vi "ImageFileOpenwithIMAQ-U16.vi"(1 "type":u32, 2 "image filepath":path=path "I:/160830- miura/20 um beads/nonsheet/160903/test2_00004.png") -> (0 "output array":u16[][](array[numeric]))   [LabVIEW 2018]
uses:
  <vilib>/Utility/file.llb/Read Delimited Spreadsheet (DBL).vi
panel:
  out "file path for TPEF 2":path=path "C:/Users/Mikami/Desktop/test.bmp"
  out "result string":string="png"
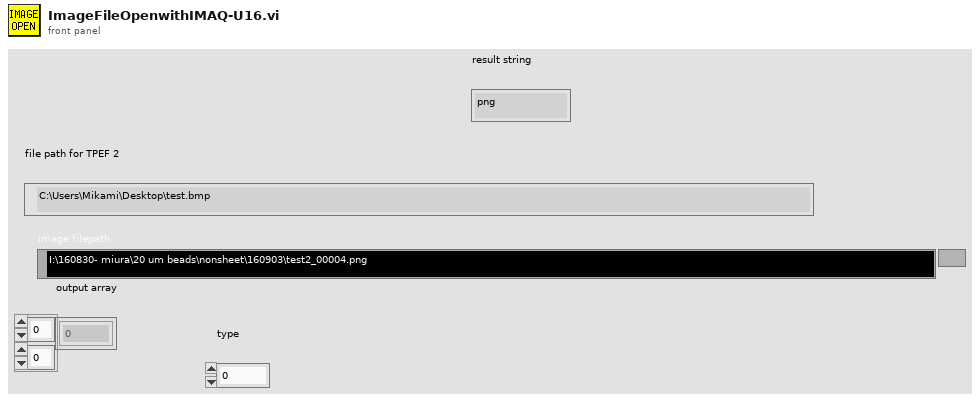
[diagram p1: front panel]
types:
  T1 = typedef "imagedata.ctl" = cluster{"image type":i32, "image depth":i32, "image":u8[], "mask":u8[], "colors":u32[], "Rectangle":cluster{"left":i16, "top":i16, "right":i16, "bottom":i16}}
  T2 = typedef "Image Type" = u32
  T3 = typedef "IMAQ Image.ctl" = refnum<image>
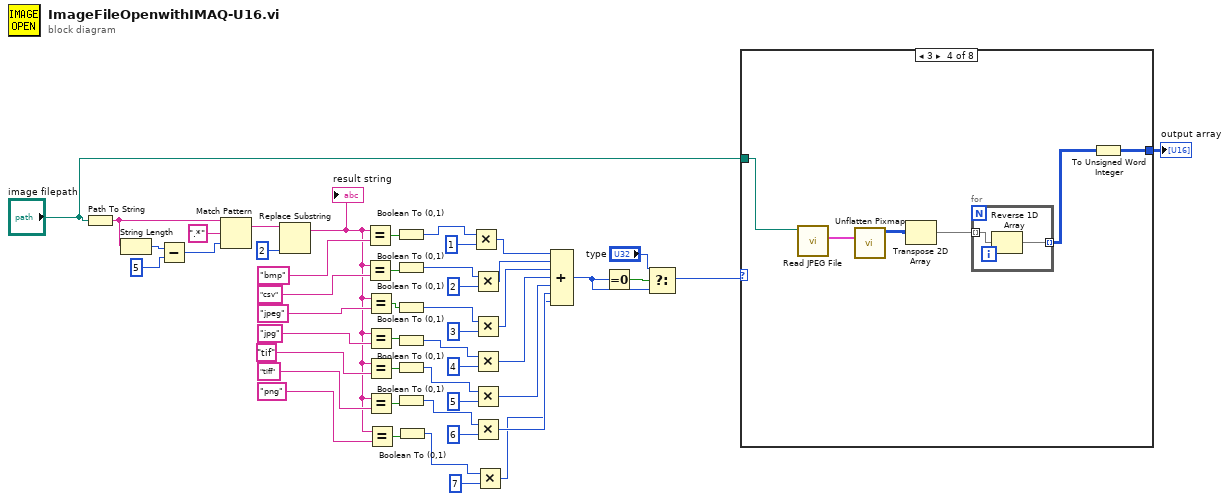
[diagram p0: block diagram]
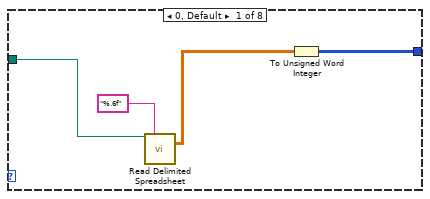
[diagram p2: hidden frame]
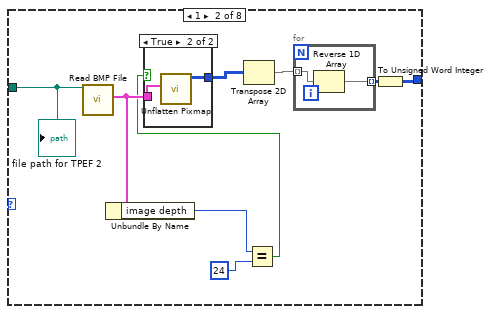
[diagram p3: hidden frame]
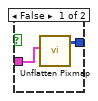
[diagram p4: hidden frame]
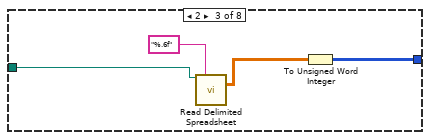
[diagram p5: hidden frame]
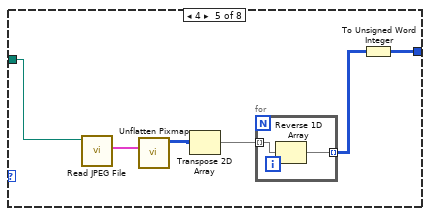
[diagram p6: hidden frame]
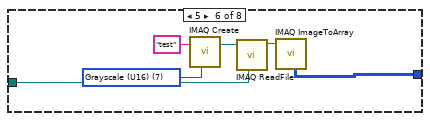
[diagram p7: hidden frame]
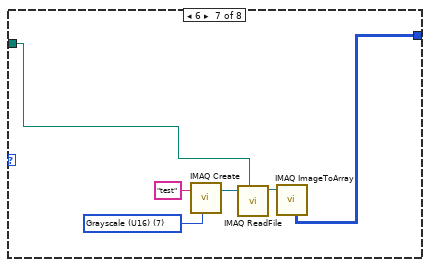
[diagram p8: hidden frame]
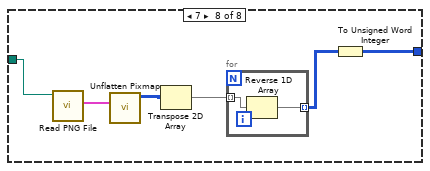
[diagram p9: hidden frame]
diagram:
  n1 = Path To String(path="image filepath") -> (string=w48:string)
  n2 = String Length(string=w48) -> (length=w47:i32)
  n3 = Subtract(x=w47, y=5) -> (x-y=w45:i32)
  n4 = Match Pattern(string=w48, regular expression=".*", offset (0)=w45) -> (match substring=w44:string)  [unwired: 3 out]
  n5 = Replace Substring(2:2 ("length (len. of substring)"), 5:w44) -> (1:w6:string)  [unwired: 2 in, 1 out]
  "result string" <- w6
  n6 = Equal?(x=w6, y="bmp" ("regular expression")) -> (x = y?=w30:bool)
  n7 = Equal?(x=w6, y="csv" ("regular expression")) -> (x = y?=w24:bool)
  n8 = Equal?(x=w6, y="jpeg" ("regular expression")) -> (x = y?=w25:bool)
  n9 = Equal?(x=w6, y="jpg" ("regular expression")) -> (x = y?=w28:bool)
  n10 = Equal?(x=w6, y="tif" ("regular expression")) -> (x = y?=w26:bool)
  n11 = Equal?(x=w6, y="tiff" ("regular expression")) -> (x = y?=w27:bool)
  n12 = Equal?(x=w6, y="png" ("regular expression")) -> (x = y?=w11:bool)
  n13 = Boolean To (0,1)(Boolean=w30) -> (0, 1=w29:i16)
  n14 = Boolean To (0,1)(Boolean=w24) -> (0, 1=w23:i16)
  n15 = Boolean To (0,1)(Boolean=w25) -> (0, 1=w22:i16)
  n16 = Boolean To (0,1)(Boolean=w28) -> (0, 1=w21:i16)
  n17 = Boolean To (0,1)(Boolean=w26) -> (0, 1=w20:i16)
  n18 = Boolean To (0,1)(Boolean=w27) -> (0, 1=w19:i16)
  n19 = Boolean To (0,1)(Boolean=w11) -> (0, 1=w9:i16)
  n20 = Multiply(x=w29, y=u8 1) -> (x*y=w18:i16)
  n21 = Multiply(x=w23, y=i8 2) -> (x*y=w17:i16)
  n22 = Multiply(x=w22, y=i8 3) -> (x*y=w16:i16)
  n23 = Multiply(x=w21, y=i8 4) -> (x*y=w15:i16)
  n24 = Multiply(x=w20, y=i8 5) -> (x*y=w14:i16)
  n25 = Multiply(x=w19, y=i8 6) -> (x*y=w13:i16)
  n26 = Multiply(x=w9, y=i8 7) -> (x*y=w8:i16)
  n27 = Compound Arithmetic op=ADD(w18, w17, w16, w15, w14, w13, w8) -> (w2:i16)
  n28 = Equal To 0?(x=w2) -> (x = 0?=w4:bool)
  n29 = Select(t="type", s=w4, f=w2) -> (s? t:f=w5:u32)
  n30 = case shown="3" w5 {
    tunnel: "image filepath" -> [w52 w62 w71 w75 w83 w90 w96 w103]
    tunnel: [w50 w54 w69 w73 w81 w89 w95 w101] -> w1
    frame 0, Default {
      n31 = call-poly <vilib>:"Read Delimited Spreadsheet.vi"("file path (dialog if empty)"=w52, "format (%.3f)"="%.6f") -> ("all rows"=w51:dbl[][])  [unwired: 8 in, 5 out]
      n32 = To Unsigned Word Integer(number=w51) -> (unsigned 16bit integer=w50:u16[][])
    }
    frame 1 {
      n33 = call <vilib>:"Read BMP File.vi"("path to BMP file"=w62) -> ("image data"=w58:T1)  [unwired: 8 in, 2 out]
      n34 = Unbundle By Name(w58) -> ("image depth"=w57:i32)
      n35 = Equal?(x=w57, y=24) -> (x = y?=w55:bool)
      n36 = case shown="True" w55 {
        tunnel: [w63 w66] -> w61
        tunnel: w58 -> [w64 w65]
        frame False {
          n37 = call <vilib>:"Unflatten Pixmap.vi"("image data"=w64) -> ("8-bit pixmap"=w63:u8[][])  [unwired: 4 in, 6 out]
        }
        frame True {
          n38 = call <vilib>:"Unflatten Pixmap.vi"("image data"=w65) -> ("24-bit pixmap"=w66:u32[][])  [unwired: 4 in, 6 out]
        }
      }
      n39 = Transpose 2D Array(2D array=w61) -> (transposed array=w60:u32[][])
      n40 = for {
        tunnel: w60 -> [w68] mode=indexing
        tunnel: [w67] -> w59 mode=indexing
        n41 = Reverse 1D Array(array=w68) -> (reversed array=w67:u32[])
      }
      n42 = To Unsigned Word Integer(number=w59) -> (unsigned 16bit integer=w54:u16[][])
      "file path for TPEF 2" <- w62
    }
    frame 2 {
      n43 = call-poly <vilib>:"Read Delimited Spreadsheet.vi"("file path (dialog if empty)"=w71, "format (%.3f)"="%.6f") -> ("all rows"=w72:dbl[][])  [unwired: 8 in, 5 out]
      n44 = To Unsigned Word Integer(number=w72) -> (unsigned 16bit integer=w69:u16[][])
    }
    frame 3 {
      n45 = call <vilib>:"Read JPEG File.vi"("path to JPEG file"=w75) -> ("image data"=w76:T1)  [unwired: 8 in, 2 out]
      n46 = call <vilib>:"Unflatten Pixmap.vi"("image data"=w76) -> ("24-bit pixmap"=w78:u32[][])  [unwired: 4 in, 6 out]
      n47 = Transpose 2D Array(2D array=w78) -> (transposed array=w77:u32[][])
      n48 = for {
        tunnel: w77 -> [w80] mode=indexing
        tunnel: [w79] -> w74 mode=indexing
        n49 = Reverse 1D Array(array=w80) -> (reversed array=w79:u32[])
      }
      n50 = To Unsigned Word Integer(number=w74) -> (unsigned 16bit integer=w73:u16[][])
    }
    frame 4 {
      n51 = call <vilib>:"Read JPEG File.vi"("path to JPEG file"=w83) -> ("image data"=w84:T1)  [unwired: 8 in, 2 out]
      n52 = call <vilib>:"Unflatten Pixmap.vi"("image data"=w84) -> ("24-bit pixmap"=w86:u32[][])  [unwired: 4 in, 6 out]
      n53 = Transpose 2D Array(2D array=w86) -> (transposed array=w85:u32[][])
      n54 = for {
        tunnel: w85 -> [w88] mode=indexing
        tunnel: [w87] -> w82 mode=indexing
        n55 = Reverse 1D Array(array=w88) -> (reversed array=w87:u32[])
      }
      n56 = To Unsigned Word Integer(number=w82) -> (unsigned 16bit integer=w81:u16[][])
    }
    frame 5 {
      w91 = T2 7 items=["Grayscale (U8)", "Grayscale (I16)", "Grayscale (SGL)", "Complex (CSG)", "RGB (U32)", "HSL (U32)", "RGB (U64)", "Grayscale (U16)"] ("Image Type")
      n57 = call "IMAQ Create"("Image Name"="test", "Image Type"=w91) -> ("New Image"=w93:T3)  [unwired: 3 in, 1 out]
      n58 = call "IMAQ ReadFile"("File Path"=w90, "Image"=w93) -> ("Image Out"=w94:T3)  [unwired: 5 in, 4 out]
      n59 = call "IMAQ ImageToArray"("Image"=w94) -> ("Image Pixels (U16)"=w89:u16[][])  [unwired: 3 in, 4 out]
    }
    frame 6 {
      w100 = T2 7 items=["Grayscale (U8)", "Grayscale (I16)", "Grayscale (SGL)", "Complex (CSG)", "RGB (U32)", "HSL (U32)", "RGB (U64)", "Grayscale (U16)"] ("Image Type")
      n60 = call "IMAQ Create"("Image Name"="test", "Image Type"=w100) -> ("New Image"=w98:T3)  [unwired: 3 in, 1 out]
      n61 = call "IMAQ ReadFile"("File Path"=w96, "Image"=w98) -> ("Image Out"=w97:T3)  [unwired: 5 in, 4 out]
      n62 = call "IMAQ ImageToArray"("Image"=w97) -> ("Image Pixels (U16)"=w95:u16[][])  [unwired: 3 in, 4 out]
    }
    frame 7 {
      n63 = call <vilib>:"Read PNG File.vi"("path to PNG file"=w103) -> ("image data"=w104:T1)  [unwired: 8 in, 2 out]
      n64 = call <vilib>:"Unflatten Pixmap.vi"("image data"=w104) -> ("24-bit pixmap"=w106:u32[][])  [unwired: 4 in, 6 out]
      n65 = Transpose 2D Array(2D array=w106) -> (transposed array=w105:u32[][])
      n66 = for {
        tunnel: w105 -> [w108] mode=indexing
        tunnel: [w107] -> w102 mode=indexing
        n67 = Reverse 1D Array(array=w108) -> (reversed array=w107:u32[])
      }
      n68 = To Unsigned Word Integer(number=w102) -> (unsigned 16bit integer=w101:u16[][])
    }
  }
  "output array" <- w1
